vi "Init Interaction.vi"(6 "Register for events? [T]":bool=TRUE, 7 "Sub Panel":refnum<vi>, 8 "error in (no error)":errorcluster, 10 "IObject":refnum<class "IObject.lvclass">) -> (0 "error out":errorcluster, 1 "Interaction Splitter Resize":refnum<user-event>, 2 "Interaction Splitter Resize":refnum<event-registration>, 3 "Interaction out":refnum<class "Interaction.lvclass">)   [LabVIEW 2013, in "Interaction.lvclass"]
doc: "Copyright 2018, Wiebe Walstra, wiebe@carya.nl."
uses:
  Interaction.lvclass
  IObject.lvclass
  Interaction.lvclass/Interaction.ctl
  IContainer.lvclass
  Interaction Splitter.lvclass
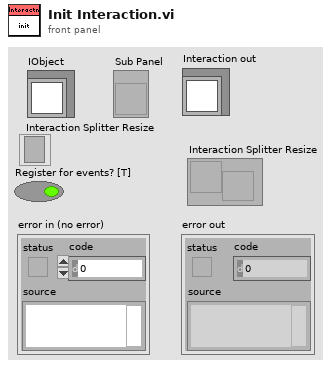
[diagram p1: front panel]
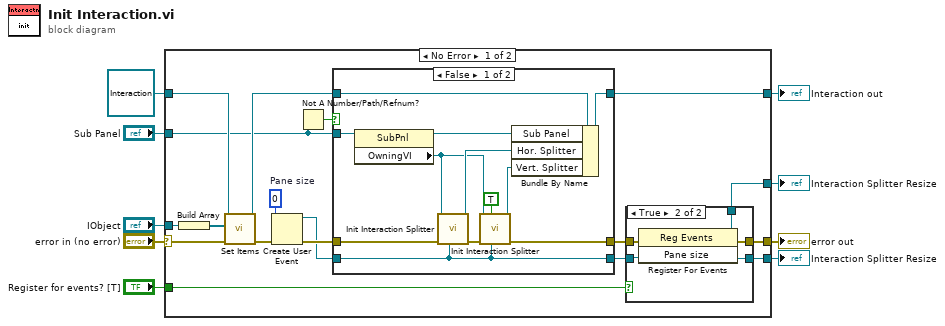
[diagram p0: block diagram]
diagram:
  n1 = case shown="No Error" "error in (no error)" {
    selector: "error in (no error)" -> [w27 w50]
    tunnel: [w18 w50] -> w8
    tunnel: [w23 w49] -> w6
    tunnel: refnum<class "Interaction.lvclass"> refnum ("Interaction in") -> [w14 w49]
    tunnel: "IObject" -> [w26 _]
    tunnel: "Sub Panel" -> [w13 _]
    tunnel: [w17 _] -> w3
    tunnel: [w10 _] -> w2
    tunnel: "Register for events? [T]" -> [w15 _]
    frame No Error {
      w21 = 0  # Pane size
      n2 = Build Array(w26) -> (w25:refnum<class "IObject.lvclass">[])
      n3 = call "Set Items.vi"("error in (no error)"=w27, "Items"=w25, "IContainer in"=w14) -> ("error out"=w20:errorcluster, "IContainer out"=w24:refnum<class "Interaction.lvclass">)  [unwired: 7 in]
      n4 = Create User Event(user event datatype=w21, error in=w20) -> (user event=w16:refnum<user-event>, error out=w19:errorcluster)
      n5 = Not A Number/Path/Refnum?(number/path/refnum=w13) -> (NaN/Path/Refnum?=w12:bool)
      n6 = case shown="False" w12 {
        tunnel: w24 -> [w30 w42]
        tunnel: [w39 w42] -> w23
        tunnel: [w36 w41] -> w22
        tunnel: w19 -> [w33 w41]
        tunnel: w16 -> [w28 w40]
        tunnel: w13 -> [w31 _]
        tunnel: [w28 w40] -> w11
        frame False {
          n7 = property class="SubPnl"(reference=w31) -> (reference out=w29:refnum<vi>, "OwningVI"=w32:refnum<vi>)  [unwired: 1 in, 1 out]
          n8 = call "Init Interaction Splitter.vi"("user event out"=w28, "error in (no error)"=w33, "Host VI"=w32) -> ("error out"=w37:errorcluster, "Interaction Splitter out"=w35:refnum<class "Interaction Splitter.lvclass">)  [unwired: 7 in]
          n9 = call "Init Interaction Splitter.vi"("user event out"=w28, "Vertical? [F]"=TRUE, "error in (no error)"=w37, "Host VI"=w32) -> ("error out"=w36:errorcluster, "Interaction Splitter out"=w38:refnum<class "Interaction Splitter.lvclass">)  [unwired: 6 in]
          n10 = Bundle By Name(cluster=w30, "Sub Panel"=w29, "Hor. Splitter"=w35, "Vert. Splitter"=w38) -> (w39:refnum<class "Interaction.lvclass">)
        }
        frame True {
        }
      }
      n11 = case shown="True" w15 {
        tunnel: w22 -> [w44 w48]
        tunnel: [w44 w47] -> w18
        tunnel: [_ w46] -> w17
        tunnel: w11 -> [w43 w45]
        tunnel: [w43 w45] -> w10
        frame False {
        }
        frame True {
          n12 = register-events(error in=w48, w45) -> (reference out=w46:refnum<event-registration>, error out=w47:errorcluster)  [unwired: 1 in]
        }
      }
    }
    frame Error {
    }
  }
  "error out" <- w8
  "Interaction out" <- w6
  "Interaction Splitter Resize" <- w3
  "Interaction Splitter Resize" <- w2
